vi "createArray_MR1.vi"(6 "Start freq":dbl, 9 "Freq step":i32=100000 format="%.2e", 10 "End freq":dbl, 11 "Shuffle?":bool) -> (3 "Riffled {X}":dbl[](array[numeric]))   [LabVIEW 2017]
uses:
  <vilib>/Analysis/1siggen.llb/Ramp Pattern by Samples.vi
  <vilib>/Analysis/1siggen.llb/Riffle Array (DBL).vi
  <vilib>/Analysis/NI_AALBase.lvlib
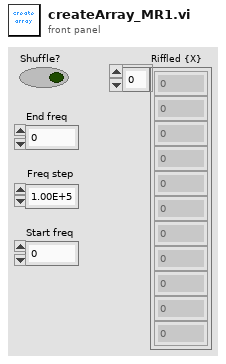
[diagram p1: front panel]
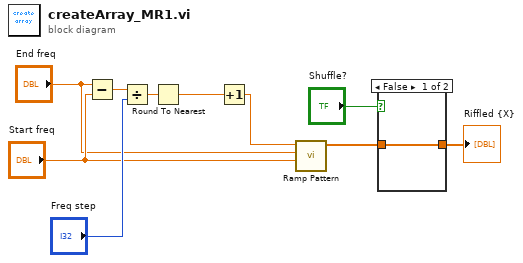
[diagram p0: block diagram]
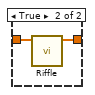
[diagram p2: hidden frame]
diagram:
  n1 = Subtract(x="End freq", y="Start freq") -> (x-y=w5:dbl)
  n2 = Divide(x=w5, y="Freq step") -> (x/y=w7:dbl)
  n3 = Round To Nearest(number=w7) -> (nearest integer value=w1:dbl)
  n4 = Increment(x=w1) -> (x+1=w2:dbl)
  n5 = call-poly <vilib>:"Ramp Pattern.vi"("start"="Start freq", "end"="End freq", "samples"=w2) -> ("Ramp Pattern"=w8:dbl[])  [unwired: 7 in, 1 out]
  n6 = case shown="False" "Shuffle?" {
    tunnel: w8 -> [w11 w13]
    tunnel: [w11 w12] -> w9
    frame False {
    }
    frame True {
      n7 = call-poly <vilib>:"Riffle.vi"("X"=w13) -> ("Riffled {X}"=w12:dbl[])  [unwired: 8 in, 2 out]
    }
  }
  "Riffled {X}" <- w9
